vi "Create Session.vi"(8 "error in (no error)":errorcluster, 10 "Close Notifier":refnum<notifier>) -> (0 "error out":errorcluster, 3 "Unit Of Work out":refnum<class "Unit Of Work Session.lvclass">)   [LabVIEW 2020, in "Conditu2.lvlib" / "Unit Of Work Session.lvclass"]
uses:
  Unit Of Work Session.lvclass
  Ref Data.ctl
  Entity Class Map.ctl
  Entity ID.ctl
  Entity/Entity.lvclass
  Unit Of Work Session.lvclass/Unit Of Work Session.ctl
  Conditu2.lvlib
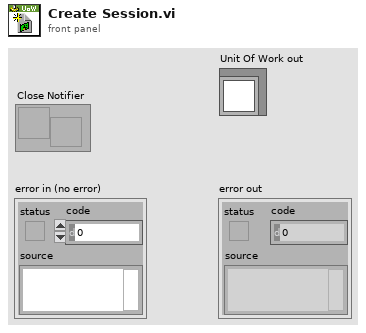
[diagram p1: front panel]
types:
  T1 = typedef "Conditu2.lvlib/Unit Of Work Session.lvclass/Ref Data.ctl" = cluster{"Entity Class Map":T2}
  T2 = typedef "Conditu2.lvlib/Unit Of Work Session.lvclass/Entity Class Map.ctl" = map{string, map{T3, refnum<class "Entity.lvclass">}}
  T3 = typedef "Conditu2.lvlib/Entity ID.ctl" = i64
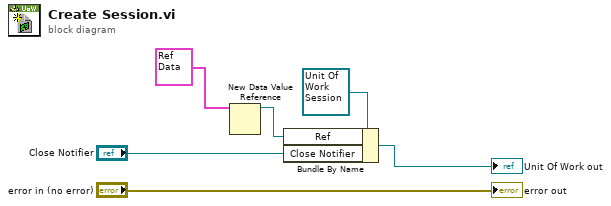
[diagram p0: block diagram]
diagram:
  n1 = New Data Value Reference(data value=T1 {"Entity Class Map"={}} ("Ref Data")) -> (data value reference=w3:refnum<data-value>)  [unwired: 1 in, 1 out]
  n2 = Bundle By Name(cluster=refnum<class "Unit Of Work Session.lvclass"> refnum ("Unit Of Work in"), "Ref"=w3, "Close Notifier"="Close Notifier") -> (→"Unit Of Work out":refnum<class "Unit Of Work Session.lvclass">)
  "error out" <- "error in (no error)"
